vi "Fs and Ns for integer periods.vi"(10 "f_integer":dbl, 11 "Fs":dbl) -> (2 "#s_integer":dbl, 3 "Fs_integer":dbl)   [LabVIEW 2013]
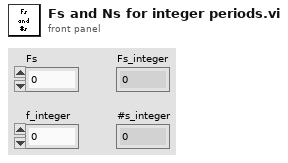
[diagram p1: front panel]
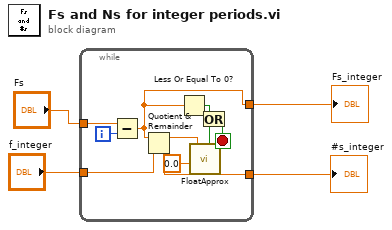
[diagram p0: block diagram]
diagram:
  n1 = while {
    tunnel: "Fs" -> [w14]
    tunnel: [w10] -> w2
    tunnel: "f_integer" -> [w8]
    tunnel: [w9] -> w1
    i -> [w13]
    stop <- w11 stop-if-true
    n2 = Subtract(x=w14, y=w13) -> (x-y=w10:dbl)
    n3 = Quotient & Remainder(x=w10, y=w8) -> (x-y*floor(x/y)=w6:dbl, floor(x/y)=w9:dbl)
    n4 = Less Or Equal To 0?(x=w10) -> (x <= 0?=w12:bool)
    n5 = call "FloatApprox.vi"("y"=0.0, "x"=w6) -> ("x ~ y?"=w5:bool)  [unwired: 2 in]
    n6 = Or(x=w12, y=w5) -> (x .or. y?=w11:bool)
  }
  "Fs_integer" <- w2
  "#s_integer" <- w1
